vi "end timer Read.vi"(4 "error in (no error)":errorcluster, 6 "Container State":T5, 7 "Display State In":T1={"Z_Source"={"connect"=FALSE, "Z_Source"=enum."initialize", "Z_State_heating"=enum."on"}, "Write"=FALSE, "Z1_ind"=0, "button state"=enum."init", "reset_timer"=FALSE, "load_timer"=FALSE, "end_timer"=TRUE}) -> (0 "error out":errorcluster, 2 "Value":bool, 3 "Display State Out":T1={"Z_Source"={"connect"=FALSE, "Z_Source"=enum."initialize", "Z_State_heating"=enum."on"}, "Write"=FALSE, "Z1_ind"=0, "button state"=enum."init", "reset_timer"=FALSE, "load_timer"=FALSE, "end_timer"=TRUE})   [LabVIEW 2019, in "Heating.lvlib" / "Z_OnSwitch.xctl"]
uses:
  Z_OnSwitch.xctl
  <vilib>/_xctls/Container State.ctl
  State.ctl
  Z_source.ctl
  Z_State.ctl
  On_ButtonState.ctl
  <vilib>/_xctls/XControlSupport.lvlib
  Heating.lvlib
panel:
  # "Replace the Value Indicator below with an Indicator of desired type.\nDo not remove this Indicator or the others from the connector pane. \nDo not change the connector pane pattern.\nThe Value Indicator should always be the second terminal from top on the output side in the connector pane."
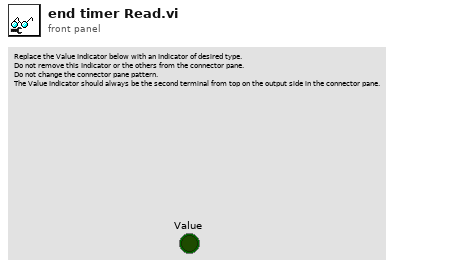
[diagram p1: front panel]
types:
  T1 = typedef "Heating.lvlib/Z_OnSwitch.xctl/State.ctl" = cluster{"Z_Source":cluster{"connect":bool, "Z_Source":T2, "Z_State_heating":T3}, "Write":bool, "Z1_ind":u8, "button state":T4, "reset_timer":bool, "load_timer":bool, "end_timer":bool}
  T2 = typedef "Heating.lvlib/Z_source.ctl" = enum8{"initialize", "local disabled", "local hand", "hand", "auto", "dist"}
  T3 = typedef "Heating.lvlib/Z_State.ctl" = enum8{"initialization", "alarm", "disabled", "not ready", "stop ready", "reserv", "switched off", "reserv2", "switched on", "check", "on min", "decrease out", "on", "increase out", "on max"}
  T4 = typedef "Heating.lvlib/Z_OnSwitch.xctl/On_ButtonState.ctl" = enum16{"init", "not connect", "local disabled", "local hand", "switch off", "off", "switch on", "on", "auto", "dist"}
  T5 = typedef "XControlSupport.lvlib/Container State.ctl" = cluster{"Indicator?":bool, "Run Mode?":bool, " Refnum":refnum<vi>}
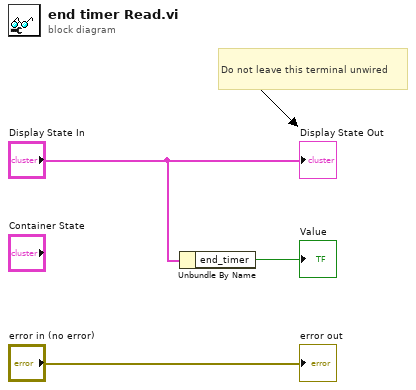
[diagram p0: block diagram]
diagram:
  # "Do not leave this terminal unwired"
  n1 = Unbundle By Name("Display State In") -> ("end_timer"=→"Value":bool)
  "error out" <- "error in (no error)"
  "Display State Out" <- "Display State In"
